vi "ReadSpeedM1.vi"(0 "VISA Refnum in":refnum<visa-resource-name>, 3 "error in (no error)":errorcluster) -> (1 "EncCnt":u32, 5 "Status":u8, 6 "VISA Refnum out":refnum<visa-resource-name>, 7 "Valid":bool, 10 "error out":errorcluster)   [LabVIEW 2015, in "Ion Motion Roboclaw.lvlib"]
uses:
  <instrlib>/Ion Motion Roboclaw/Ion Motion Roboclaw.lvlib
panel:
  in  "Address":u8
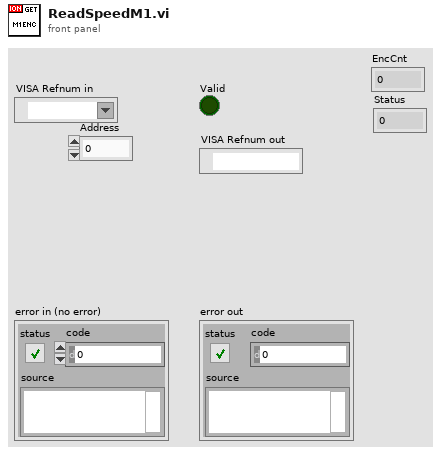
[diagram p1: front panel]
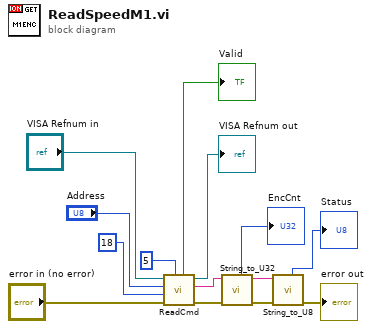
[diagram p0: block diagram]
diagram:
  n1 = call <instrlib>:"ReadCmd.vi"("Read Count"=u32 5, "error in (no error)"="error in (no error)", "Cmd"=u8 18, "Address"="Address", "VISA Refnum in"="VISA Refnum in") -> ("error out"=w9:errorcluster, "Output"=w8:string, "VISA Refnum out"=→"VISA Refnum out":refnum<visa-resource-name>, "Valid"=→"Valid":bool)  [unwired: 3 in]
  n2 = call <instrlib>:"String_to_U32.vi"("error in (no error)"=w9, "String"=w8) -> ("error out"=w13:errorcluster, "rest of the binary string"=w14:string, "number"=→"EncCnt":u32)  [unwired: 5 in]
  n3 = call <instrlib>:"String_to_U8.vi"("error in (no error)"=w13, "String"=w14) -> ("error out"=→"error out":errorcluster, "Argument"=→"Status":u8)  [unwired: 5 in, 1 out]
